vi "Configure test.vi"(6 "Assert VI Path":path, 7 "Existing Queue Elements":string, 8 "error in (no error)":errorcluster, 11 "Basic Str Starts With in":refnum<class "Str Starts With.lvclass">) -> (0 "error out":errorcluster, 3 "Basic Str Starts With out":refnum<class "Str Starts With.lvclass">)   [LabVIEW 2018, in "Str Starts With.lvclass"]
uses:
  Str Starts With.lvclass
  <vilib>/Utility/Data Type/Type Definitions/Data Type.ctl
  9ee76486-a755-4515-9fb4-fb1f1c61538e.vi
  <vilib>/JDP Science/JSONtext/Find Item.vi
  9ee76486-a755-4515-9fb4-fb1f1c61538e.vi/171a7b55-6f4b-4348-b9c4-e97a8e549e53.vi
  9ee76486-a755-4515-9fb4-fb1f1c61538e.vi/47dd8245-1aa2-432e-892a-b711c0c9e0fa.vi
  <vilib>/JDP Science/JSONtext/String Subset.vi
  Test Class String IDs.vi
  <vilib>/JDP Science/JSONtext/Parsing/Parse Full Path or Item Name.vi
  <vilib>/JDP Science/JSONtext/Offset/Find Item Locations by Path.vi
  <vilib>/JDP Science/JSONtext/JSON text to Variant.vi
  <vilib>/JDP Science/JSONtext/Variant to JSON Text.vi
  <vilib>/JDP Science/JSONtext/Set Item.vi
  String.lvclass
  Test.lvclass
  <vilib>/Utility/Data Type/NI_Data Type.lvlib
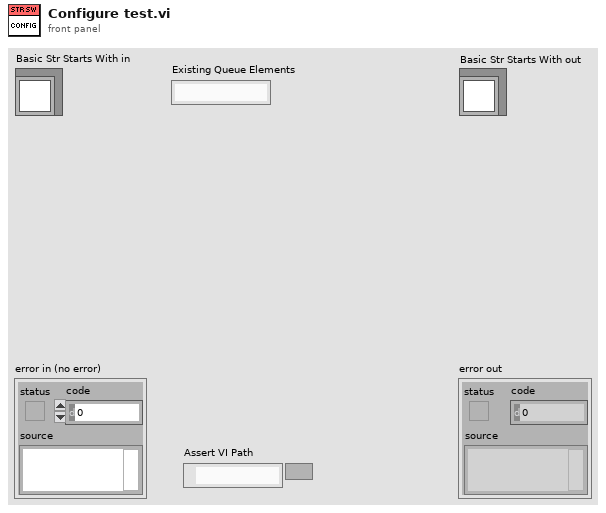
[diagram p1: front panel]
types:
  T1 = typedef "NI_Data Type.lvlib/Data Type.ctl" = enum8{"Invalid Type", "Void", "I8", "I16", "I32", "I64", "U8", "U16", "U32", "U64", "Single Float", "Double Float", "Extended Float", "Single Complex", "Double Complex", "Extended Complex", "Enum U8", "Enum U16", "Enum U32", "Enum U64", "Single Float With Unit", "Double Float With Unit", "Extended Float With Unit", "Single Complex with Unit", "Double Complex with Unit", "Extended Complex with Unit", "Boolean", "String", "Path", "Picture", "Tag", "Array", "Cluster", "Variant", "LV Variant", "Waveform", "Timestamp", "Digital Waveform", "Digital Data", "ExpressData", "Refnum", "External Data", "VI", "Poly VI", "LabVIEW Class Instance", "Fixed Point"}
  T2 = cluster{"Additional Data":string, "Comparison Value":string, "Invert?":string, "Assert Name":string, "Comment":string, "Default Failure Action":string, "Assert Build Timestamp":string, "Assert Builder User Name":string, "Data Type":string, "Assert VI Name":string, "Evaluation String":string}
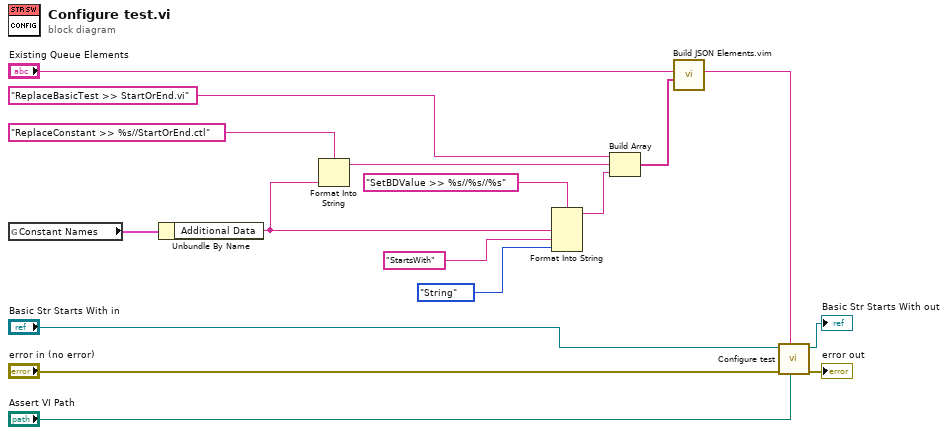
[diagram p0: block diagram]
diagram:
  n1 = global read "Test Class String IDs.vi" "Constant Names"() -> (w7:T2)
  n2 = Unbundle By Name(w7) -> ("Additional Data"=w6:string)
  n3 = Format Into String(format string="ReplaceConstant >> %s//StartOrEnd.ctl" ("Append Element(s)"), w6) -> (resulting string=w8:string)  [unwired: 2 in, 1 out]
  n4 = Format Into String(format string="SetBDValue >> %s//%s//%s", w6, "StartsWith" ("input 2"), Data_Type."String" ("input 3")) -> (resulting string=w10:string)  [unwired: 2 in, 1 out]
  n5 = Build Array("ReplaceBasicTest >> StartOrEnd.vi" ("Append Element(s)"), w8, w10) -> (w2:string[])
  n6 = call "Build JSON Elements.vim"("Append Element(s)"=w2, "JSON Elements in ({})"="Existing Queue Elements") -> ("JSON Elements out"=w1:string)  [unwired: 9 in]
  n7 = call-parent "Configure test.vi"("Assert VI Path"="Assert VI Path", "Existing Queue Elements"=w1, "error in (no error)"="error in (no error)", "Basic String in"="Basic Str Starts With in") -> ("error out"=→"error out":errorcluster, "Basic String out"=→"Basic Str Starts With out":refnum<class "Str Starts With.lvclass">)  [unwired: 6 in]
